vi "Send UpdateCamTestEvents.vi"(7 "Message Priority (Normal)":T8=enum."Normal", 8 "error in (no error)":errorcluster, 10 "CameraTestingEvnt":T1, 11 "Message Enqueuer":refnum<class "Message Enqueuer.lvclass">) -> (0 "error out":errorcluster, 3 "Message Enqueuer out":refnum<class "Message Enqueuer.lvclass">)   [LabVIEW 2020, in "ICameraTestingUI.lvlib" / "UpdateCamTestEvents Msg.lvclass"]
doc: "This VI sends the message to an actor."
uses:
  UpdateCamTestEvents Msg.lvclass
  <vilib>/ActorFramework/Message Enqueuer/Message Enqueuer.lvclass
  <vilib>/ActorFramework/Message Enqueuer/Message Priority.ctl
  ICameraTesting/ICameraTesting/TypeDef/Events.ctl
  Camera/ICamera/ICamera/TypeDef/SnapInfo.ctl
  ICameraTesting/ICameraTesting/TypeDef/FrameRateValReceived.ctl
  ICameraTesting/ICameraTesting/TypeDef/ImgTypeValReceived.ctl
  ICameraTesting/ICameraTesting/TypeDef/ResolutionValReceived.ctl
  ICameraTesting/ICameraTesting/TypeDef/VideoOptCodesUpdated.ctl
  ICameraTesting/ICameraTesting/TypeDef/VideoOptionsInfo.ctl
  ICameraTesting/ICameraTesting/TypeDef/StatusLogUpdate.ctl
  C:/Program Files (x86)/National Instruments/LabVIEW 2020/vi.lib/ActorFramework/Message/Message.lvclass
  UpdateCamTestEvents Msg.lvclass/UpdateCamTestEvents Msg.ctl
  <vilib>/ActorFramework/Message Enqueuer/Message Enqueuer.lvclass/Message Enqueuer.ctl
  <vilib>/ActorFramework/Message Priority Queue/Priority Enqueue.vi
  Camera/ICamera/ICamera/ICamera.lvclass
  ICameraTesting/ICameraTesting/ICameraTesting.lvclass
  ICameraTesting/ICameraTesting/TypeDef/VideoBufferUpdate.ctl
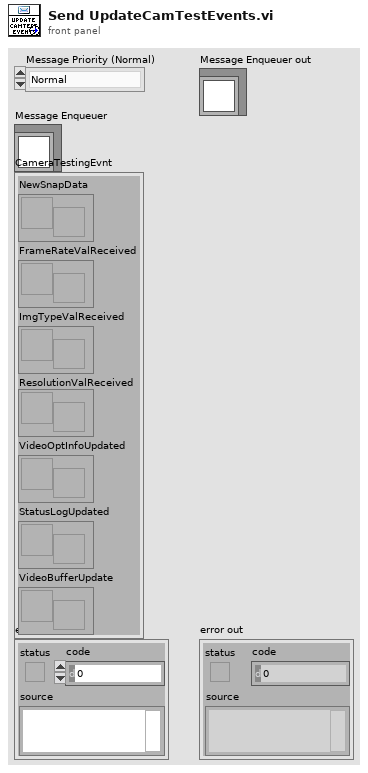
[diagram p1: front panel]
types:
  T1 = typedef "ICameraTesting.lvlib/ICameraTesting.lvclass/Events.ctl" = cluster{"NewSnapData":refnum<user-event>, "FrameRateValReceived":T2, "ImgTypeValReceived":T3, "ResolutionValReceived":T4, "VideoOptInfoUpdated":T5, "StatusLogUpdated":T6, "VideoBufferUpdate":T7}
  T2 = typedef "ICameraTesting.lvlib/ICameraTesting.lvclass/FrameRateValReceived.ctl" = refnum<user-event>
  T3 = typedef "ICameraTesting.lvlib/ICameraTesting.lvclass/ImgTypeValReceived.ctl" = refnum<user-event>
  T4 = typedef "ICameraTesting.lvlib/ICameraTesting.lvclass/ResolutionValReceived.ctl" = refnum<user-event>
  T5 = typedef "ICameraTesting.lvlib/ICameraTesting.lvclass/VideoOptCodesUpdated.ctl" = refnum<user-event>
  T6 = typedef "ICameraTesting.lvlib/ICameraTesting.lvclass/StatusLogUpdate.ctl" = refnum<user-event>
  T7 = typedef "ICameraTesting.lvlib/ICameraTesting.lvclass/VideoBufferUpdate.ctl" = refnum<user-event>
  T8 = typedef "Actor Framework.lvlib/Message Enqueuer.lvclass/Message Priority.ctl" = enum16{"Low", "Normal", "High"}
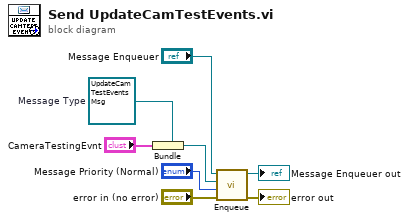
[diagram p0: block diagram]
diagram:
  w5 = refnum<class "UpdateCamTestEvents Msg.lvclass"> refnum  # Message Type
  n1 = Bundle(cluster=w5, "CameraTestingEvnt") -> (w4:refnum<class "UpdateCamTestEvents Msg.lvclass">)
  n2 = call <vilib>:"Enqueue.vi"("error in (no error)"="error in (no error)", "Message Priority (Normal)"="Message Priority (Normal)", "Message"=w4, "Message Enqueuer in"="Message Enqueuer") -> ("error out"=→"error out":errorcluster, "Message Enqueuer out"=→"Message Enqueuer out":refnum<class "Message Enqueuer.lvclass">)  [unwired: 6 in]
